vi "UpdateLaserStatus.vi"(8 "error in (no error)":errorcluster, 10 "event data":cluster{"Label":string, "Visable?":bool}, 11 "LaserController in":refnum<class "LaserController.lvclass">) -> (0 "error out":errorcluster, 3 "LaserController out":refnum<class "LaserController.lvclass">)   [LabVIEW 2020, in "LaserController.lvlib" / "LaserController.lvclass"]
uses:
  LaserController.lvclass
  LaserController.lvclass/LaserController.ctl
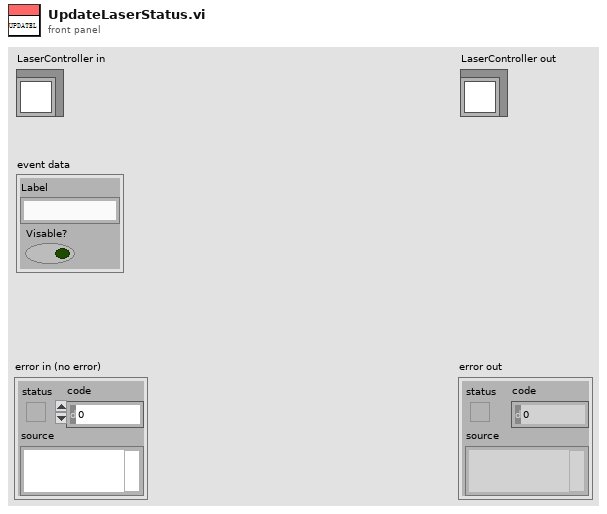
[diagram p1: front panel]
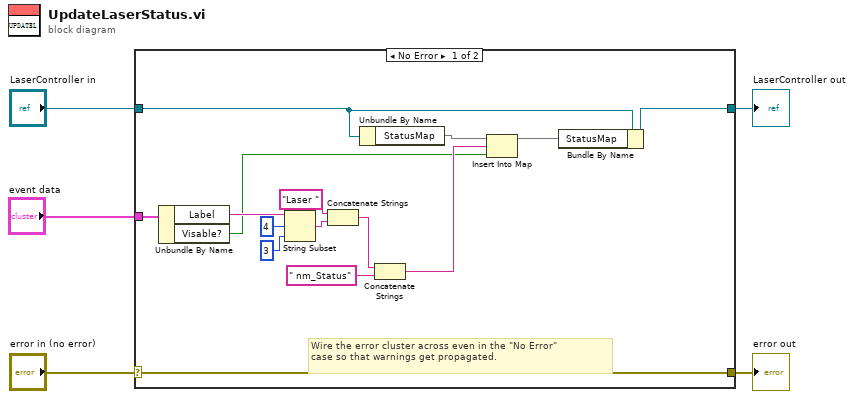
[diagram p0: block diagram]
diagram:
  n1 = case shown="No Error" "error in (no error)" {
    selector: "error in (no error)" -> [w20 w22]
    tunnel: [w20 w22] -> w4
    tunnel: [w17 w21] -> w2
    tunnel: "LaserController in" -> [w18 w21]
    tunnel: "event data" -> [w19 _]
    frame No Error {
      # "Wire the error cluster across even in the \"No Error\"\ncase so that warnings get propagated."
      n2 = Unbundle By Name(w19) -> ("Label"=w12:string, "Visable?"=w6:bool)
      n3 = String Subset(string=w12, offset (0)=4, length (rest)=3 ("length (rest)")) -> (substring=w13:string)
      n4 = Concatenate Strings("Laser " ("string"), w13) -> (w10:string)
      n5 = Unbundle By Name(w18) -> ("StatusMap"=w9:map{string, bool})
      n6 = Concatenate Strings(w10, " nm_Status" ("Key")) -> (w7:string)
      n7 = Insert Into Map(map in=w9, key=w7, value=w6) -> (map out=w8:map{string, bool})  [unwired: 2 out]
      n8 = Bundle By Name(cluster=w18, "StatusMap"=w8) -> (w17:refnum<class "LaserController.lvclass">)
    }
    frame Error {
    }
  }
  "error out" <- w4
  "LaserController out" <- w2
